vi "Get Field Refnums.vi"(8 "error in (no error)":errorcluster, 11 "Basic Form in":refnum<class "Basic Form.lvclass">) -> (0 "error out":errorcluster, 2 "Field Refnums":map{string, refnum<vi>}(c390), 3 "Basic Form out":refnum<class "Basic Form.lvclass">)   [LabVIEW 2020, in "Form.lvlib" / "Basic Form.lvclass"]
uses:
  Basic Form.lvclass
  C:/Users/User/Desktop/Raman Program/Database OOP/source/Database OOP/Table Libraries/Basic Table/Basic Table Class/Basic Table.lvclass
  Basic Form.lvclass/Basic Form.ctl
  Column Libraries/Field Interfaces/Field Interface Class/Field Interface.lvclass
  Basic Table/Basic Table Class/Basic Table.lvclass
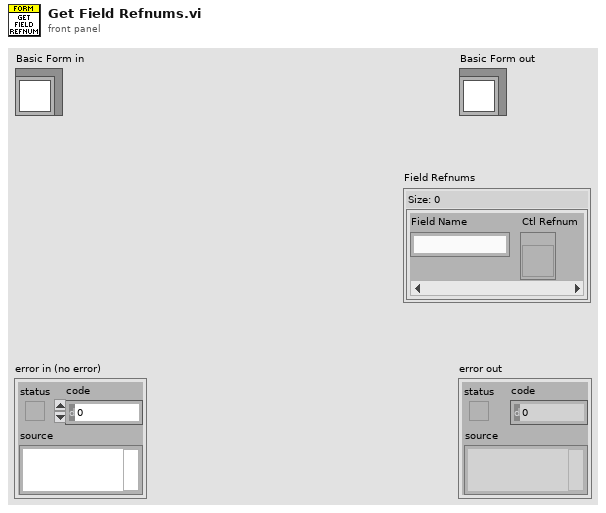
[diagram p1: front panel]
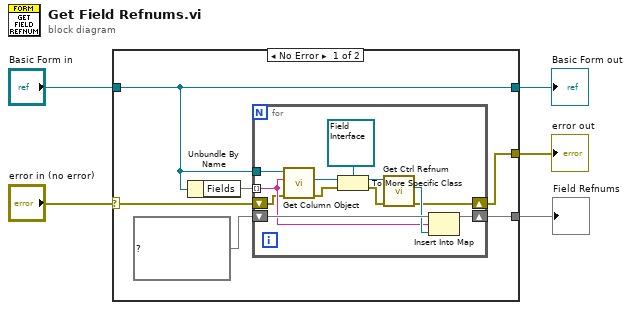
[diagram p0: block diagram]
diagram:
  n1 = case shown="No Error" "error in (no error)" {
    selector: "error in (no error)" -> [w8 w25]
    tunnel: [w7 w25] -> w4
    tunnel: [w10 w24] -> w2
    tunnel: "Basic Form in" -> [w10 w24]
    tunnel: [w6 _] -> w1
    frame No Error {
      n2 = Unbundle By Name(w10) -> ("Fields"=w11:set{string})
      n3 = for {
        tunnel: w11 -> [w14] mode=indexing
        tunnel: w10 -> [w18]
        shift-right: [w16] -> w6
        shift-left: map{string, refnum<vi>} {} ("Field Refnums") -> [w17]
        shift-right: [w13] -> w7
        shift-left: w8 -> [w12]
        n4 = call "Get Column Object.vi"("error in (no error)"=w12, "Column Name"=w14, "Table in"=w18) -> ("error out"=w21:errorcluster, "Column Object"=w19:refnum<class "Column Interface.lvclass">)  [unwired: 6 in, 1 out]
        n5 = To More Specific Class(target class=refnum<class "Field Interface.lvclass"> refnum ("Field Interfaces.lvlib:Field Interface.lvclass"), reference=w19, error in=w21) -> (specific class reference=w23:refnum<class "Field Interface.lvclass">, error out=w20:errorcluster)
        n6 = call-dynamic "Get Ctrl Refnum.vi"("error in (no error)"=w20, "Field Interface in"=w23) -> ("error out"=w13:errorcluster, "Ctl Refnum"=w15:refnum<vi>)  [unwired: 7 in, 1 out]
        n7 = Insert Into Map(map in=w17, key=w14, value=w15) -> (map out=w16:map{string, refnum<vi>})  [unwired: 2 out]
      }
    }
    frame Error {
    }
  }
  "error out" <- w4
  "Basic Form out" <- w2
  "Field Refnums" <- w1
